vi "RequestAndTrace.vi"(0 "JSONRef in":T1, 1 "TraceRef":refnum<vi>, 5 "method":string, 7 "params":variant, 11 "error in (no error)":errorcluster) -> (4 "JSONRef out":T1, 6 "reponse":string, 15 "error out":errorcluster)   [LabVIEW 2017]
uses:
  jsonRPCwebservice/client/reference.ctl
  <vilib>/httpClient/ClientHandle.ctl
  jsonRPCwebservice/client/Request_int_str.vi
  jsonRPCwebservice/client/JSON_RPC_client.lvlib
  <vilib>/httpClient/LabVIEWHTTPClient.lvlib
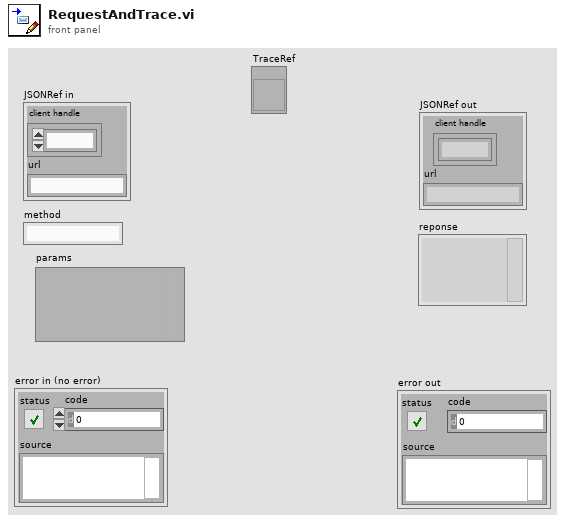
[diagram p1: front panel]
types:
  T1 = typedef "JSON_RPC_client.lvlib/reference.ctl" = cluster{"client handle":T2, "url":string}
  T2 = typedef "LabVIEWHTTPClient.lvlib/ClientHandle.ctl" = refnum<k1>
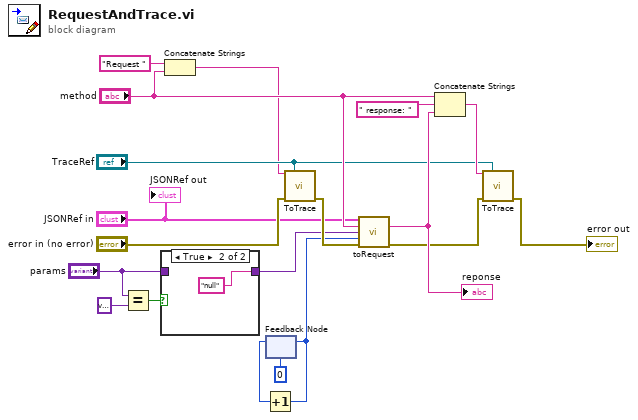
[diagram p0: block diagram]
diagram:
  n1 = Equal?(x="params", y=variant) -> (x = y?=w3:bool)
  n2 = case shown="True" w3 {
    tunnel: "params" -> [w20 _]
    tunnel: [w20 "null"] -> w1
    frame False {
    }
    frame True {
    }
  }
  n3 = Concatenate Strings("Request ", "method") -> (w12:string)
  n4 = feedback #1(0 ("id")) -> (w6:i32)
  n5 = Increment(x=w6) -> (x+1=w5:i32)
  n6 = feedback-in #1(w5) -> ()
  n7 = call "ToTrace.vi"("ToTrace"=w12, "TraceRef"="TraceRef", "error in (no error)"="error in (no error)") -> ("error out"=w10:errorcluster)  [unwired: 12 in]
  n8 = call-poly "toRequest.vi"("reference in"="JSONRef in", "method"="method", "params"=w1, "id"=w5, "error in (no error)"=w10) -> ("response"=w18:string, "error out"=w14:errorcluster)  [unwired: 8 in, 1 out]
  "reponse" <- w18
  n9 = Concatenate Strings("method", " response: " ("string"), w18) -> (w19:string)
  n10 = call "ToTrace.vi"("ToTrace"=w19, "TraceRef"="TraceRef", "error in (no error)"=w14) -> ("error out"=→"error out":errorcluster)  [unwired: 12 in]
  "JSONRef out" <- "JSONRef in"
